vi "prepareDish.vi"(8 "error in (no error)":errorcluster, 10 "appliance":refnum<class "Appliance.lvclass">, 11 "Kitchen in":refnum<class "Kitchen.lvclass">) -> (0 "error out":errorcluster, 3 "Kitchen out":refnum<class "Kitchen.lvclass">)   [LabVIEW 2011, in "Kitchen.lvclass"]
uses:
  Kitchen.lvclass
  Appliance/Appliance.lvclass
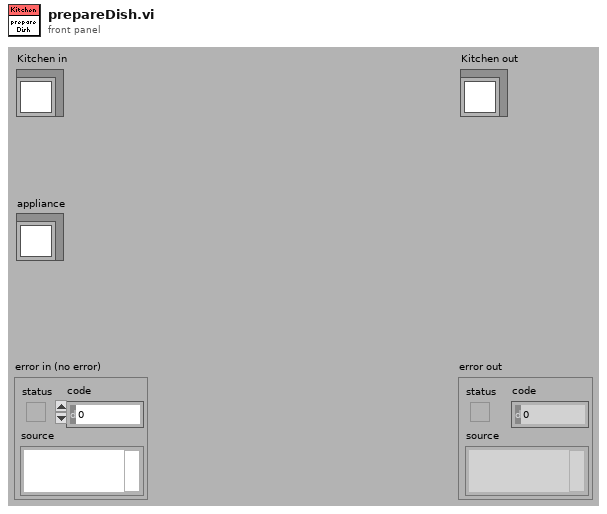
[diagram p1: front panel]
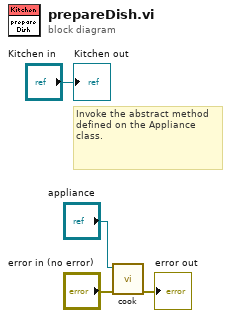
[diagram p0: block diagram]
diagram:
  # "Invoke the abstract method defined on the Appliance class."
  n1 = call "cook.vi"("error in (no error)"="error in (no error)", "Appliance in"="appliance") -> ("error out"=→"error out":errorcluster)  [unwired: 8 in, 1 out]
  "Kitchen out" <- "Kitchen in"
